vi "Show Tree Snippet.vi"() -> ()   [LabVIEW 2017, in "Tree API.lvlib" / "Tree.lvclass"]
doc: "Recursively traverse down wired Tree ID and populate the Tree Control with the contents of the Tree.\n\nBecause the Tree Control requires to have only one root element, the Root ID has to be specified. This means that if you have multiple roots in your Tree you need to visualize them seperately."
uses:
  Tree.lvclass
panel:
  in  "Tree Reference":refnum<vi>
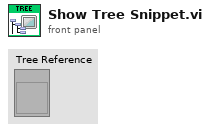
[diagram p1: front panel]
types:
  T1 = cluster{"Left Cell String":string, "Child Text":string[], "Child Tag":string, "Item Indent":i32, "Child Only?":bool, "Glyph Index":i32}[]
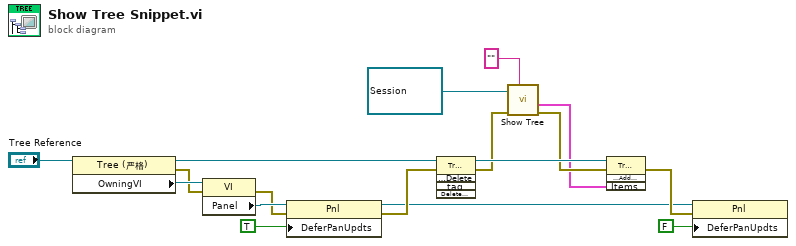
[diagram p0: block diagram]
diagram:
  n1 = property class="Tree (严格)"(reference="Tree Reference") -> (reference out=w13:refnum<vi>, error out=w16:errorcluster, "OwningVI"=w17:refnum<vi>)  [unwired: 1 in]
  n2 = property class="VI"(reference=w17, error in=w16) -> (error out=w14:errorcluster, "Panel"=w15:refnum<vi>)  [unwired: 1 out]
  n3 = property class="Pnl"(reference=w15, error in=w14, "DeferPanUpdts"=TRUE ("Defer Panel Updates")) -> (reference out=w7:refnum<vi>, error out=w12:errorcluster)
  n4 = invoke class="Tree (strict)" method="Edit Tree Items.Delete"(reference=w13, error in=w12) -> (reference out=w9:refnum<vi>, error out=w5:errorcluster)  [unwired: 3 in, 3 out]
  n5 = call "Show Tree.vi"("Root ID"="", "Error In"=w5, "Tree"=refnum<data-value> refnum) -> ("Error Out"=w4:errorcluster, "Items Out"=w3:T1)  [unwired: 6 in, 1 out]
  n6 = invoke class="Tree (strict)" method="Edit Tree Items.Add Multiple Items to End"(reference=w9, error in=w4, "Items"=w3) -> (error out=w8:errorcluster)  [unwired: 1 in, 3 out]
  n7 = property class="Pnl"(reference=w7, error in=w8, "DeferPanUpdts"=FALSE ("Defer Panel Updates")) -> ()  [unwired: 2 out]
